vi "parseConfigData.vi"(8 "error in (no error)":errorcluster, 11 "results-JSON string":string) -> (0 "error out":errorcluster, 3 "Data out":T1={"CenterWavelength"=0.0, "ChipHSpacing"="$.configuration", "ChipHeight"="$.configuration", "ChipName"="$.configuration", "ChipSerialNumber"="$.configuration", "ChipVSpacing"="$.configuration", "ChipWidth"="$.configuration", "DeviceType"="$.configuration", "FitParameters"=[], "Gains"=[], "HardwareAvgAvailable"="$.configuration"})   [LabVIEW 2023, in "CCD.lvclass"]
uses:
  CCD.lvclass
  Config.ctl
  Gain.ctl
  41762e30-eae5-4a4c-8725-288ba60ead02.vi
  <vilib>/JDP Science/JSONtext/Next JSON Value.vi
  <vilib>/JDP Science/JSONtext/String Subset.vi
  <vilib>/JDP Science/JSONtext/Parsing/Advance past next JSON Value (inlined COPY).vi
  <vilib>/JDP Science/JSONtext/Parsing/Advance past whitespace.vi
  <vilib>/JDP Science/JSONtext/Parsing/Advance past String.vi
  <vilib>/JDP Science/JSONtext/Parsing/Advance past Number.vi
  <vilib>/JDP Science/JSONtext/Parsing/Advance past Line Ending.vi
  <vilib>/JDP Science/JSONtext/Parsing/Parse Full Path or Item Name.vi
  <vilib>/JDP Science/JSONtext/Parsing/Advance past Array.vi
  <vilib>/JDP Science/JSONtext/Parsing/Advance past Object.vi
  <vilib>/JDP Science/JSONtext/support/Error Cluster From Code.vi
  <vilib>/JDP Science/JSONtext/Offset/Find Item Locations by Path.vi
  <vilib>/JDP Science/JSONtext/JSON text to Variant.vi
  <vilib>/JDP Science/JSONtext/LVClass Serializer/JSONtext LVClass Serializer.lvclass
  CCD.lvclass/CCD.ctl
  <vilib>/JDP Science/JSONtext/JSONtext.lvlib
panel:
  in  "Token":i32
  # "Connector Pane"
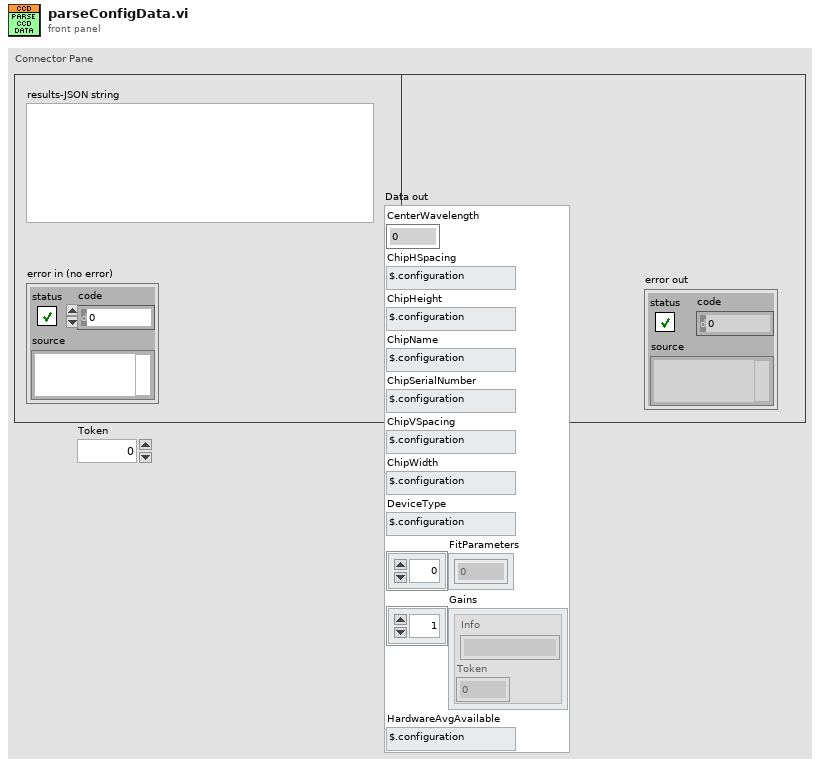
[diagram p1: front panel]
types:
  T1 = typedef "CCD.lvclass/Config.ctl" = cluster{"CenterWavelength":dbl, "ChipHSpacing":string, "ChipHeight":string, "ChipName":string, "ChipSerialNumber":string, "ChipVSpacing":string, "ChipWidth":string, "DeviceType":string, "FitParameters":dbl[], "Gains":T2[], "HardwareAvgAvailable":string}
  T2 = typedef "CCD.lvclass/Gain.ctl" = cluster{"Info":string, "Token":u16}
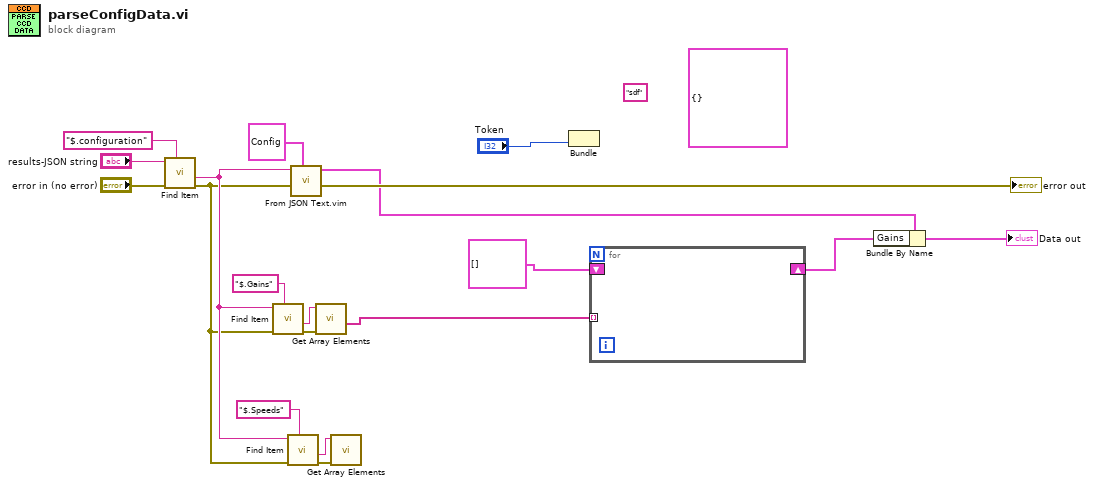
[diagram p0: block diagram]
diagram:
  (unwired) cluster{} {}
  (unwired) "sdf" ("Info")
  n1 = call <vilib>:"Find Item.vi"("$Path or Item Name"="$.configuration", "error in (no error)"="error in (no error)", "JSON"="results-JSON string") -> ("error out"=w10:errorcluster, "<JSON>"=w11:string)  [unwired: 5 in, 2 out]
  n2 = call <vilib>:"Find Item.vi"("$Path or Item Name"="$.Gains", "error in (no error)"=w10, "JSON"=w11) -> ("error out"=w9:errorcluster, "<JSON>"=w8:string)  [unwired: 5 in, 2 out]
  n3 = call <vilib>:"Find Item.vi"("$Path or Item Name"="$.Speeds", "error in (no error)"=w10, "JSON"=w11) -> ("error out"=w13:errorcluster, "<JSON>"=w12:string)  [unwired: 5 in, 2 out]
  n4 = call "From JSON Text.vim"("Data Type and Default Value"=T1 {"CenterWavelength"=0.0, "ChipHSpacing"="", "ChipHeight"="", "ChipName"="$.configuration", "ChipSerialNumber"="$.configuration", "ChipVSpacing"="$.configuration", "ChipWidth"="$.configuration", "DeviceType"="$.configuration", "FitParameters"=[], "Gains"=[], "HardwareAvgAvailable"="$.configuration"} ("Gain"), "error in (no error)"=w10, "JSON"=w11) -> ("error out"=→"error out":errorcluster, "Data out"=w4:T1)  [unwired: 7 in]
  n5 = call <vilib>:"Get Array Elements.vi"("error in (no error)"=w9, "JSON"=w8) -> ("<JSON>"=w6:string[])  [unwired: 7 in, 2 out]
  n6 = call <vilib>:"Get Array Elements.vi"("error in (no error)"=w13, "JSON"=w12) -> ()  [unwired: 7 in, 3 out]
  n7 = Bundle("Token"="Token") -> ()  [unwired: 2 in, 1 out]
  n8 = for {
    tunnel: w6 -> [w20] mode=indexing
    shift-right: [_] -> w3
    shift-left: T2[] [] ("Array") -> [_]
  }
  n9 = Bundle By Name(cluster=w4, "Gains"=w3) -> (→"Data out":T1)
